vi "TB-Update Moving Average.vi"(1 "state in":T1, 2 "fine":dbl, 5 "SPL":dbl, 11 "error in (no error)":errorcluster) -> (3 "state out":T1, 8 "moving average":dbl, 15 "error out":errorcluster)   [LabVIEW 2020]
uses:
  Typedefs/TB-Runtime state.ctl
  <vilib>/sound2/lvsound2.llb/Sound File Refnum.ctl
  Typedefs/TB-Setup Log.ctl
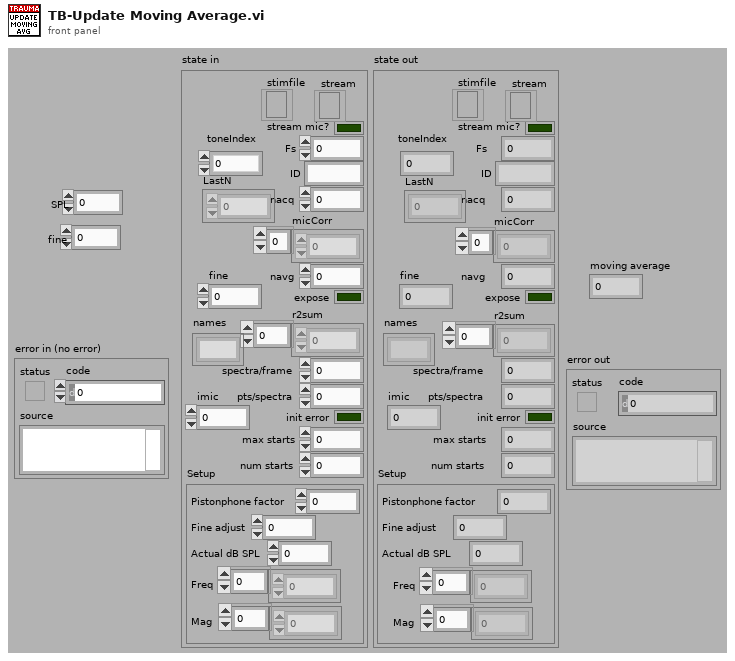
[diagram p1: front panel]
types:
  T1 = typedef "TB-Runtime state.ctl" = cluster{"stimfile":T2, "stream mic?":bool, "Fs":dbl, "ID":string, "micCorr":dbl[], "navg":i32, "r2sum":dbl[], "expose":bool, "spectra/frame":i32, "pts/spectra":i32, "nacq":i32, "init error":bool, "max starts":i32, "num starts":i32, "Setup":T3, "toneIndex":i32, "LastN":dbl[], "fine":dbl, "imic":i32, "stream":refnum<file>, "names":string[]}
  T2 = typedef "Sound File Refnum.ctl" = refnum<file>
  T3 = typedef "TB-Setup Log.ctl" = cluster{"Pistonphone factor":dbl, "Fine adjust":dbl, "Actual dB SPL":dbl, "Freq":dbl[], "Mag":dbl[]}
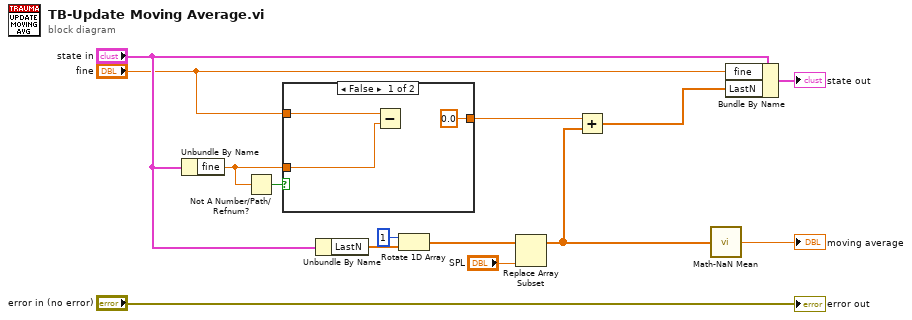
[diagram p0: block diagram]
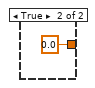
[diagram p2: hidden frame]
diagram:
  n1 = Unbundle By Name("state in") -> ("fine"=w7:dbl)
  n2 = Not A Number/Path/Refnum?(number/path/refnum=w7) -> (NaN/Path/Refnum?=w6:bool)
  n3 = case shown="False" w6 {
    tunnel: w7 -> [w16 _]
    tunnel: "fine" -> [w17 _]
    tunnel: [0.0 0.0] -> w3
    frame False {
      n4 = Subtract(x=w17, y=w16) -> ()  [unwired: 1 out]
    }
    frame True {
    }
  }
  n5 = Unbundle By Name("state in") -> ("LastN"=w12:dbl[])
  n6 = Rotate 1D Array(1:w12, 2:1 ("n")) -> (0:w4:dbl[])
  n7 = Replace Array Subset(array=w4, new element="SPL") -> (w1:dbl[])  [unwired: 1 in]
  n8 = Add(x=w3, y=w1) -> (x+y=w2:dbl[])
  n9 = call "Math-NaN Mean.vi"("Array"=w1) -> ("NaN Mean"=→"moving average":dbl)
  n10 = Bundle By Name(cluster="state in", "fine"="fine", "LastN"=w2) -> (→"state out":T1)
  "error out" <- "error in (no error)"
